vi "PIM Evaluate Measurement.vi"(7 "Current Count":dbl=1.0, 8 "Measurement Results":T11 {"IMPower_dBc(s)" format="%.2f"; "TxFreqs" format="%.2f"; "IMFreq(s)" format="%.2f"; "IMPower(s)" format="%.2f"; "TxPower" format="%.2f"}, 9 "PIM Test Parameters":T1={"Stimulus"={"C1 Pwr dBm"=0.0, "C2 Pwr dBm"=0.0, "Power Units"=enum."dBm", "Meas Type"=enum."Time", "C1 Freq MHz"=0.0, "C2 Freq MHz"=0.0, "Swept Freq Step"=0}, "Measure"={"IM Order"=0, "Direction"=0, "Averaging"=1, "ALC ON?"=TRUE, "Peak Hold?"=TRUE, "Peak last N"=1, "Ref Level dBm"=-100.0, "Ref Units"=enum."dBm", "Num Samples"=1, "Sample units"=enum."Sample(s)", "Update Rate (s)"=0.0, "DUT PORT"=enum."Port 1", "Percent (%)"=100}, "Display"={"Power Scale"={"yRange_min"=0, "yRange_max"=0}, "xRange_span"=5}} {"Stimulus"."Swept Freq Step" items=[".2", ".4", "1.0", "2.0"]; "Measure"."Averaging" items=["None", "Minimum", "Normal", "High", "Maximum"]; "Measure"."Direction" items=["Reverse", "Forward", "Auxiliary"]; "Measure"."IM Order" items=["3rd", "5th", "7th", "9th", "11th", "13th", "15th", "17th", "19th", "21st", "23rd", "25th", "27th", "29th", "31st", "33rd"]}, 11 "Steps per sample":u32) -> (0 "% Passed":dbl format="%.2g", 1 "Passed Limits?":bool, 2 "Peak Value":dbl, 4 "Actual Peak Samples":i32)   [LabVIEW 2011]
uses:
  drivers/PIM/PIM Results.ctl
  TypeDefs/PIM Test Parameters.ctl
  TypeDefs/PIM Stimulus Parameters.ctl
  BPIMCore/HW IO/PIM Sweep Step Size.ctl
  TypeDefs/PIM Measurement Parameters.ctl
  BPIMCore/HW IO/IMOrder.ctl
  BPIMCore/HW IO/MeasMode.ctl
  BPIMCore/HW IO/HW Averaging.ctl
  TypeDefs/PIM Meas Units.ctl
  BPIMCore/HW IO/DUTport.ctl
  TypeDefs/PIM Display Parameters.ctl
  OpenG/array/array.llb/Filter 1D Array with Scalar (Boolean)__ogtk.vi
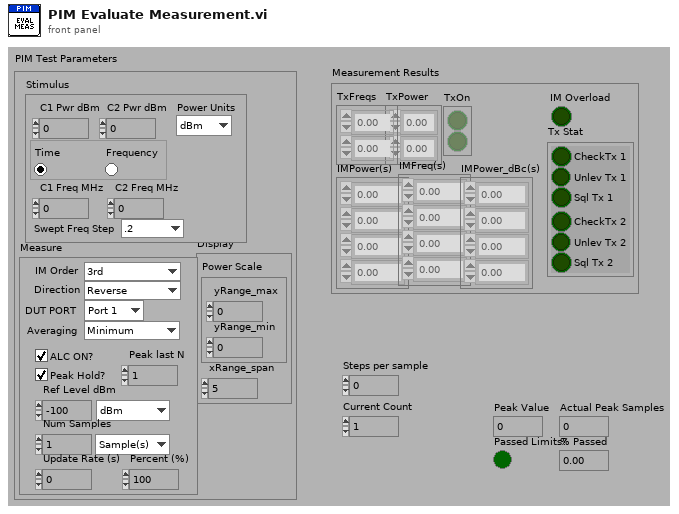
[diagram p1: front panel]
types:
  T1 = typedef "PIM Test Parameters.ctl" = cluster{"Stimulus":T2, "Measure":T4, "Display":T10}
  T2 = typedef "PIM Stimulus Parameters.ctl" = cluster{"C1 Pwr dBm":dbl, "C2 Pwr dBm":dbl, "Power Units":enum16{"dBm", "Watts"}, "Meas Type":enum32{"Time", "Frequency"}, "C1 Freq MHz":dbl, "C2 Freq MHz":dbl, "Swept Freq Step":T3}
  T3 = typedef "PIM Sweep Step Size.ctl" = u16
  T4 = typedef "PIM Measurement Parameters.ctl" = cluster{"IM Order":T5, "Direction":T6, "Averaging":T7, "ALC ON?":bool, "Peak Hold?":bool, "Peak last N":u32, "Ref Level dBm":dbl, "Ref Units":enum16{"dBm", "dBc"}, "Num Samples":u32, "Sample units":T8, "Update Rate (s)":dbl, "DUT PORT":T9, "Percent (%)":u8}
  T5 = typedef "IMOrder.ctl" = u8
  T6 = typedef "MeasMode.ctl" = u16
  T7 = typedef "HW Averaging.ctl" = u16
  T8 = typedef "PIM Meas Units.ctl" = enum16{"Sample(s)", "Second(s)", "Sweep(s)"}
  T9 = typedef "DUTport.ctl" = enum16{"Port 1", "Port 2"}
  T10 = typedef "PIM Display Parameters.ctl" = cluster{"Power Scale":cluster{"yRange_min":i32, "yRange_max":i32}, "xRange_span":u32}
  T11 = typedef "PIM Results.ctl" = cluster{"TxFreqs":dbl[], "TxPower":dbl[], "TxOn":bool[], "IMPower(s)":dbl[], "IMFreq(s)":dbl[], "Tx Stat":cluster{"CheckTx 1":bool, "Unlev Tx 1":bool, "Sql Tx 1":bool, "CheckTx 2":bool, "Unlev Tx 2":bool, "Sql Tx 2":bool}, "IM Overload":bool, "IMPower_dBc(s)":dbl[]}
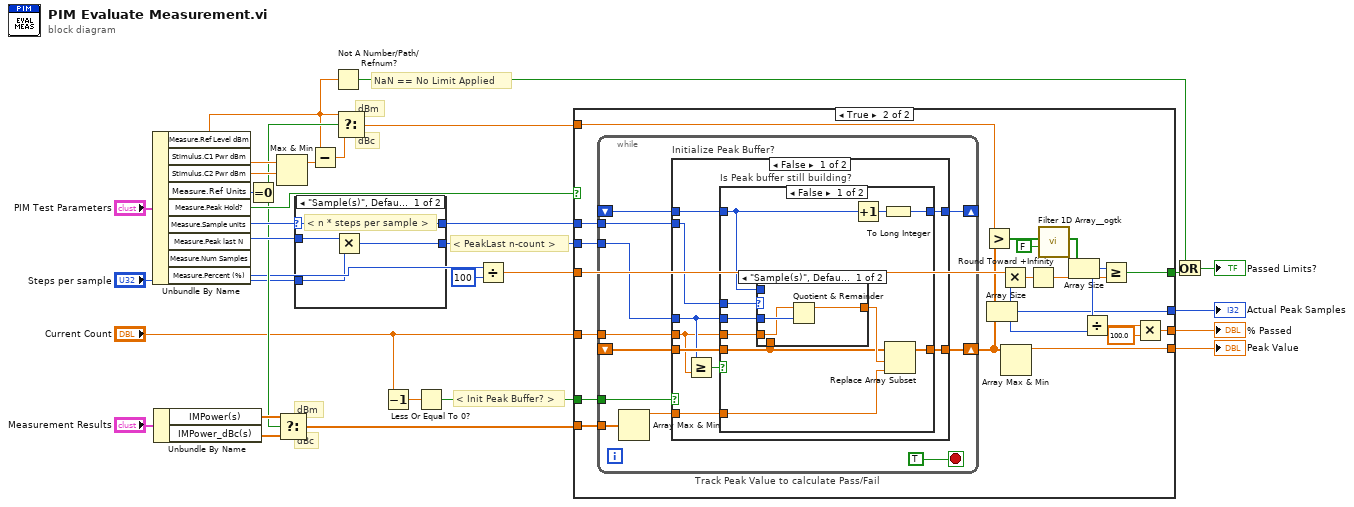
[diagram p0: block diagram]
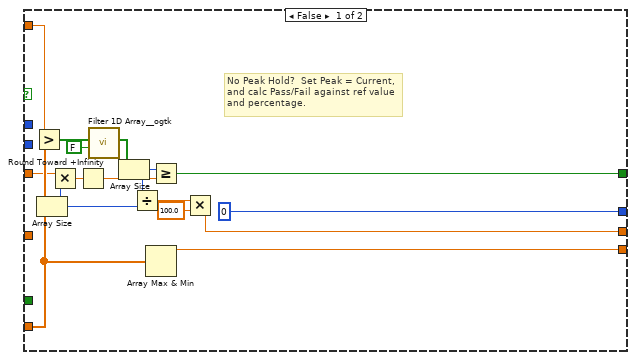
[diagram p3: hidden frame]
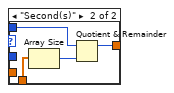
[diagram p4: hidden frame]
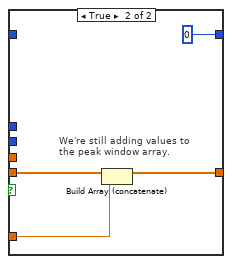
[diagram p5: hidden frame]
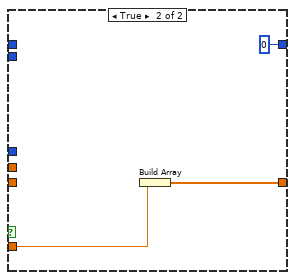
[diagram p6: hidden frame]
diagram:
  # "NaN == No Limit Applied"
  # "dBc"
  # "dBm"
  # "dBc"
  # "dBm"
  # "< Init Peak Buffer? >"
  # "< PeakLast n-count >"
  n1 = Unbundle By Name("PIM Test Parameters") -> ("Measure.Ref Level dBm"=w12:dbl, "Stimulus.C1 Pwr dBm"=w19:dbl, "Stimulus.C2 Pwr dBm"=w18:dbl, "Measure.Ref Units"=w20:enum16{"dBm", "dBc"}, "Measure.Peak Hold?"=w23:bool, "Measure.Sample units"=w30:T8, "Measure.Peak last N"=w29:u32, "Measure.Percent (%)"=w4:u8)  [unwired: 1 out]
  n2 = Unbundle By Name("Measurement Results") -> ("IMPower(s)"=w16:dbl[], "IMPower_dBc(s)"=w15:dbl[])
  n3 = Equal To 0?(x=w20) -> (x = 0?=w14:bool)
  n4 = Max & Min(x=w19, y=w18) -> (max(x,y)=w21:dbl)  [unwired: 1 out]
  n5 = Select(t=w16, s=w14, f=w15) -> (s? t:f=w13:dbl[])
  n6 = case "Samples/Seconds" shown="\"Sample(s)\", Default" w30 {
    selector: w30 -> [w33 w37]
    tunnel: w29 -> [w35 w36]
    tunnel: [w34 w36] -> w28
    tunnel: "Steps per sample" -> [w32 _]
    tunnel: [w33 w37] -> w27
    frame "Sample(s)", Default {
      # "< n * steps per sample >"
      n7 = Multiply(x=w35, y=w32) -> (x*y=w34:u32)
    }
    frame "Second(s)" {
      # "< Peak sec >"
    }
  }
  n8 = Subtract(x=w12, y=w21) -> (x-y=w22:dbl)
  n9 = Not A Number/Path/Refnum?(number/path/refnum=w12) -> (NaN/Path/Refnum?=w10:bool)
  n10 = Select(t=w12, s=w14, f=w22) -> (s? t:f=w17:dbl)
  n11 = Decrement(x="Current Count") -> (x-1=w5:dbl)
  n12 = Less Or Equal To 0?(x=w5) -> (x <= 0?=w26:bool)
  n13 = Divide(x=w4, y=u8 100) -> (x/y=w2:dbl)
  n14 = case shown="True" w23 {
    tunnel: w13 -> [w50 w73]
    tunnel: w17 -> [w53 w61]
    tunnel: [w43 w59] -> w11
    tunnel: [w52 w68] -> w25
    tunnel: w28 -> [_ w72]
    tunnel: w27 -> [_ w71]
    tunnel: "Current Count" -> [_ w70]
    tunnel: w26 -> [_ w69]
    tunnel: [0 w55] -> w24
    tunnel: w2 -> [w49 w62]
    tunnel: [w38 w54] -> w1
    frame False {
      # "No Peak Hold?  Set Peak = Current, and calc Pass/Fail against ref value\nand percentage."
      n15 = Greater?(x=w53, y=w50) -> (0:w47:bool[])
      n16 = Array Size(array=w50) -> (size(s)=w41:i32)
      n17 = Multiply(x=w49, y=w41) -> (x*y=w48:dbl)
      n18 = Round Toward +Infinity(x=w48) -> (ceil(x): smallest int >= x=w44:dbl)
      n19 = call-poly "Filter 1D Array__ogtk.vi"("items to filter"=FALSE, "array"=w47) -> ("filtered array"=w45:bool[])  [unwired: 4 in, 1 out]
      n20 = Array Size(array=w45) -> (size(s)=w42:i32)
      n21 = Divide(x=w42, y=w41) -> (x/y=w40:dbl)
      n22 = Array Max & Min(array=w50) -> (max value=w52:dbl)  [unwired: 3 out]
      n23 = Greater Or Equal?(x=w42, y=w44) -> (x >= y?=w43:bool)
      n24 = Multiply(x=w40, y=100.0) -> (x*y=w38:dbl)
    }
    frame True {
      n25 = while "Track Peak Value to calculate Pass/Fail" {
        tunnel: w73 -> [w79]
        tunnel: w72 -> [w83]
        tunnel: w71 -> [w82]
        shift-right: [w81] -> _
        shift-left: _ -> [w76]
        shift-right: [w80] -> w60
        shift-left: _ -> [w75]
        tunnel: w70 -> [w77]
        tunnel: w69 -> [w74]
        stop <- TRUE stop-if-true
        n26 = Array Max & Min(array=w79) -> (max value=w78:dbl)  [unwired: 3 out]
        n27 = case "Initialize Peak Buffer?" shown="False" w74 {
          tunnel: w83 -> [w89 _]
          tunnel: w82 -> [w85 _]
          tunnel: [w92 0] -> w81
          tunnel: [w86 w116] -> w80
          tunnel: w78 -> [w93 w115]
          tunnel: w77 -> [w88 _]
          tunnel: w76 -> [w91 _]
          tunnel: w75 -> [w90 _]
          frame False {
            n28 = Greater Or Equal?(x=w89, y=w88) -> (x >= y?=w87:bool)
            n29 = case "Is Peak buffer still building?" shown="False" w87 {
              tunnel: w93 -> [w99 w112]
              tunnel: w90 -> [w95 w114]
              tunnel: [w103 w113] -> w86
              tunnel: w89 -> [w102 _]
              tunnel: w88 -> [w100 _]
              tunnel: [w97 0] -> w92
              tunnel: w91 -> [w96 _]
              tunnel: w85 -> [w94 _]
              frame False {
                n30 = case shown="\"Sample(s)\", Default" w94 {
                  tunnel: w102 -> [w106 _]
                  tunnel: [w105 w109] -> w101
                  tunnel: w100 -> [w104 _]
                  tunnel: w96 -> [_ w107]
                  tunnel: w95 -> [_ w110]
                  frame "Sample(s)", Default {
                    n31 = Quotient & Remainder(x=w104, y=w106) -> (x-y*floor(x/y)=w105:dbl)  [unwired: 1 out]
                  }
                  frame "Second(s)" {
                    n32 = Array Size(array=w110) -> (size(s)=w108:i32)
                    n33 = Quotient & Remainder(x=w107, y=w108) -> (x-y*floor(x/y)=w109:i32)  [unwired: 1 out]
                  }
                }
                n34 = Increment(x=w96) -> (x+1=w98:i32)
                n35 = To Long Integer(number=w98) -> (32bit integer=w97:i32)
                n36 = Replace Array Subset(array=w95, new element=w99, index=w101) -> (w103:dbl[])
              }
              frame True {
                # "We're still adding values to\nthe peak window array."
                n37 = Build Array (concatenate)(w114, w112) -> (w113:dbl[])
              }
            }
          }
          frame True {
            n38 = Build Array(w115) -> (w116:dbl[])
          }
        }
      }
      n39 = Greater?(x=w61, y=w60) -> (0:w66:bool[])
      n40 = Array Size(array=w60) -> (size(s)=w55:i32)
      n41 = Multiply(x=w62, y=w55) -> (x*y=w67:dbl)
      n42 = Array Max & Min(array=w60) -> (max value=w68:dbl)  [unwired: 3 out]
      n43 = Round Toward +Infinity(x=w67) -> (ceil(x): smallest int >= x=w63:dbl)
      n44 = call-poly "Filter 1D Array__ogtk.vi"("items to filter"=FALSE, "array"=w66) -> ("filtered array"=w64:bool[])  [unwired: 4 in, 1 out]
      n45 = Array Size(array=w64) -> (size(s)=w56:i32)
      n46 = Divide(x=w56, y=w55) -> (x/y=w58:dbl)
      n47 = Greater Or Equal?(x=w56, y=w63) -> (x >= y?=w59:bool)
      n48 = Multiply(x=w58, y=100.0) -> (x*y=w54:dbl)
    }
  }
  "Peak Value" <- w25
  "Actual Peak Samples" <- w24
  "% Passed" <- w1
  n49 = Or(x=w10, y=w11) -> (x .or. y?=→"Passed Limits?":bool)
